vi "Extract Numbers with Match Pattern 2.vi"() -> ()   [LabVIEW 2020]
panel:
  out "Number":string[](array[string])
  out "Numbers":dbl[](array[numeric])
  in  "Stop Button":bool
  in  "String":string="one 2 -3 4.0 5.5"
  # "OverView :\n\nRequirements:\n\nInstructions:"
  # "Note :"
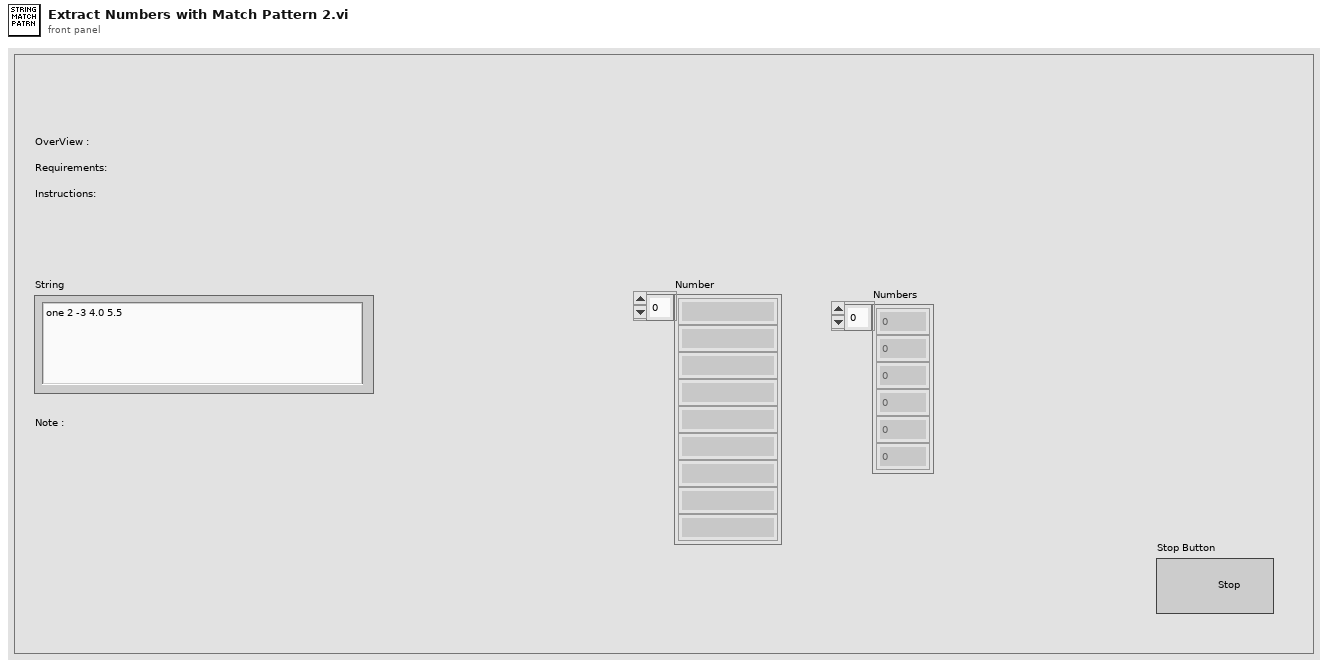
[diagram p1: front panel]
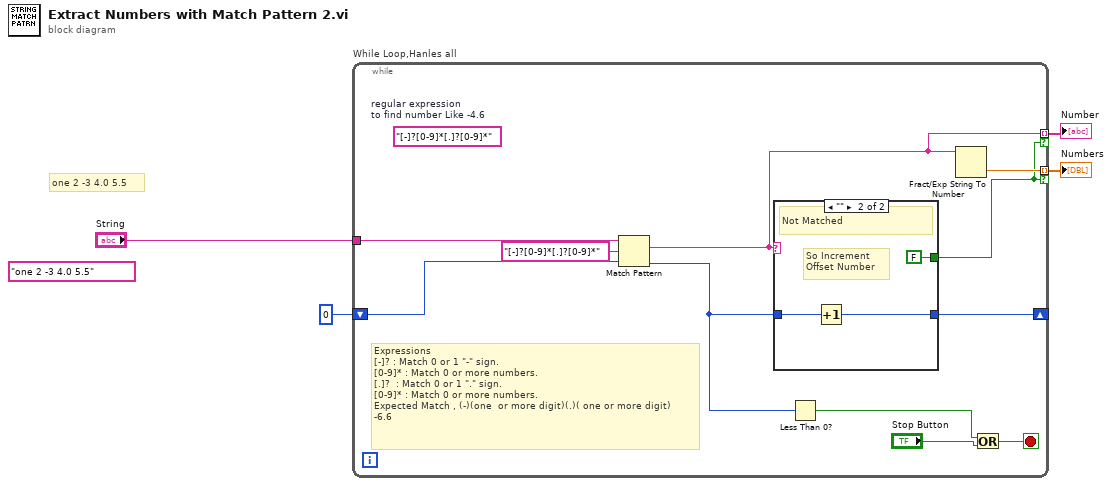
[diagram p0: block diagram]
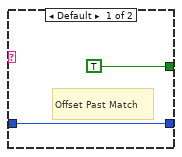
[diagram p2: hidden frame]
diagram:
  (unwired) "one 2 -3 4.0 5.5" ("String")
  # "one 2 -3 4.0 5.5"
  n1 = while "While Loop,Hanles all" {
    tunnel: "String" -> [w15]
    tunnel: [w14] -> w2 mode=indexing if=w6
    shift-right: [w12] -> _
    shift-left: 0 -> [w13]
    tunnel: [w5] -> w1 mode=indexing if=w6
    stop <- w9 stop-if-true
    (unwired) "[-]?[0-9]*[.]?[0-9]*"  # regular expression  to find number Like -4.6
    # "Expressions\n[-]? : Match 0 or 1 \"-\" sign.\n[0-9]* : Match 0 or more numbers.\n[.]?  : Match 0 or 1 \".\" sign.\n[0-9]* : Match 0 or more numbers.\nExpected Match , (-)(one  or more digit)(.)( one or more digit)\n-6.6"
    n2 = Match Pattern(string=w15, regular expression="[-]?[0-9]*[.]?[0-9]*", offset (0)=w13) -> (match substring=w5:string, offset past match=w7:i32)  [unwired: 2 out]
    n3 = case shown="\"\"" w5 {
      tunnel: w7 -> [w17 w20]
      tunnel: [w17 w19] -> w12
      tunnel: [TRUE FALSE] -> w6
      frame Default {
        # "Offset Past Match"
      }
      frame "" {
        # "So Increment \nOffset Number"
        # "Not Matched"
        n4 = Increment(x=w20) -> (x+1=w19:i32)
      }
    }
    n5 = Less Than 0?(x=w7) -> (x < 0?=w8:bool)
    n6 = Fract/Exp String To Number(string=w5) -> (number=w14:dbl)  [unwired: 3 in, 1 out]
    n7 = Or(x=w8, y="Stop Button") -> (x .or. y?=w9:bool)
  }
  "Numbers" <- w2
  "Number" <- w1
